vi "align.vi"(7 "I2C Ref Out":T1, 8 "error in (no error)":errorcluster, 11 "Angle":ext) -> (0 "error out":errorcluster, 2 "curAngle":ext, 3 "I2C Ref Out out":T1)   [LabVIEW 2017]
uses:
  <vilib>/myRIO/Instrument Drivers/Onboard IO/I2C/typedefs/I2C Reference.ctl
  <vilib>/myRIO/Common/Instrument Driver Framework/Utilities/typedefs/myRIO Generic Hardware Reference.ctl
  <vilib>/myRIO/Common/Instrument Driver Framework/Utilities/typedefs/Hardware Version Enum.ctl
  <vilib>/myRIO/Common/Instrument Driver Framework/Utilities/typedefs/myRIO v1.0 Reference.ctl
  <vilib>/myRIO/Common/Instrument Driver Framework/Utilities/typedefs/Generic FPGA Reference.ctl
  <vilib>/myRIO/Common/Instrument Driver Framework/myRIO v1.0/I2C/typedefs/I2C Channels Enum.ctl
  <vilib>/myRIO/Instrument Drivers/Onboard IO/I2C/typedefs/I2C Configuration.ctl
  <vilib>/myRIO/Instrument Drivers/Onboard IO/I2C/typedefs/I2C Transfer Rate.ctl
  <vilib>/myRIO/Instrument Drivers/Onboard IO/PWM/typedefs/PWM Reference.ctl
  <vilib>/myRIO/Common/Instrument Driver Framework/myRIO v1.0/PWM/typedefs/PWM Channels Enum.ctl
  <vilib>/myRIO/Instrument Drivers/Onboard IO/PWM/typedefs/PWM Configuration.ctl
  <vilib>/userdefined/High Color/nirio_resource_hc.ctl
  <vilib>/myRIO/Instrument Drivers/Onboard IO/DIO/typedefs/DIO Reference.ctl
  <vilib>/myRIO/Common/Instrument Driver Framework/myRIO v1.0/DIO/typedefs/DIO Channels List.ctl
  <vilib>/myRIO/Common/Instrument Driver Framework/myRIO v1.0/DIO/typedefs/DIO Channels Enum.ctl
  <vilib>/myRIO/Common/Instrument Driver Framework/Utilities/vis/Is FPGA Ref Available.vi
  <vilib>/myRIO/Common/Instrument Driver Framework/myRIO v1.0/PWM/vis/myRIO v1.1 Open PWM.vi
  <vilib>/myRIO/Instrument Drivers/Onboard IO/PWM/vis/Set Duty Cycle and Frequency.vi
  <vilib>/myRIO/Common/Instrument Driver Framework/myRIO v1.0/DIO/vis/myRIO v1.1 Open DIO.vi
  <vilib>/myRIO/Instrument Drivers/Onboard IO/DIO/vis/Write.vi
  <vilib>/myRIO/Common/Instrument Driver Framework/Utilities/vis/Validate Channels.vi
  <vilib>/myRIO/Common/Instrument Driver Framework/myRIO v1.0/PWM/vis/myRIO v1.0 Reserve PWM.vi
  <vilib>/myRIO/Common/Instrument Driver Framework/myRIO v1.0/DIO/vis/myRIO v1.0 Reserve DIO.vi
  <vilib>/myRIO/Common/Instrument Driver Framework/myRIO v1.0/PWM/vis/myRIO v1.0 Build MUX Configuration PWM.vi
  <vilib>/myRIO/Common/Instrument Driver Framework/myRIO v1.0/Resource Manager/vis/myRIO v1.0 Reserve Channel List.vi
  <vilib>/myRIO/Common/Instrument Driver Framework/myRIO v1.0/DIO/vis/myRIO v1.0 Build MUX Configuration DIO.vi
  <vilib>/myRIO/Common/Instrument Driver Framework/myRIO v1.0/Resource Manager/vis/myRIO v1.0 Create Configuration List.vi
  <vilib>/myRIO/Common/Instrument Driver Framework/myRIO v1.0/Resource Manager/vis/myRIO v1.0 Reserve Channel.vi
  <vilib>/myRIO/Common/Instrument Driver Framework/myRIO v1.0/Resource Manager/vis/myRIO v1.0 Unreserve Channel.vi
  <vilib>/myRIO/Common/Instrument Driver Framework/myRIO v1.0/Resource Manager/vis/myRIO v1.0 Build Mutex Name.vi
  <vilib>/Utility/VariantDataType/GetNumericInfo.vi
  <vilib>/Utility/error.llb/Error Cluster From Error Code.vi
  <vilib>/myRIO/Common/Instrument Driver Framework/myRIO v1.0/myRIO v1.1 Open.vi
  <vilib>/myRIO/Common/Instrument Driver Framework/Utilities/vis/IO Manager.vi
  <vilib>/myRIO/Common/Instrument Driver Framework/Utilities/vis/Configuration Manager.vi
  <vilib>/myRIO/Common/Instrument Driver Framework/myRIO v1.0/Resource Manager/vis/myRIO v1.0 Configure IO.vi
  <vilib>/myRIO/Common/Instrument Driver Framework/myRIO v1.0/myRIO v1.0 Close.vi
  <vilib>/myRIO/Common/Instrument Driver Framework/myRIO v1.0/DIO/vis/myRIO v1.0 Write DIO.vi
  <vilib>/myRIO/Common/Instrument Driver Framework/myRIO v1.0/PWM/vis/myRIO v1.0 Write PWM.vi
  <vilib>/myRIO/Express VI/Onboard IO/DO/DO Express VI.xnode
  <vilib>/myRIO/Instrument Drivers/Onboard IO/DIO/vis/myRIO DIO Open.xnode
  <vilib>/myRIO/Express VI/Onboard IO/PWM/PWM Express VI.xnode
  <vilib>/myRIO/Instrument Drivers/Onboard IO/PWM/vis/myRIO PWM Open.xnode
  <vilib>/myRIO/Instrument Drivers/Onboard IO/DIO/DIO.lvlib
  <vilib>/myRIO/Instrument Drivers/Onboard IO/PWM/PWM.lvlib
  <vilib>/myRIO/Instrument Drivers/Onboard IO/I2C/I2C.lvlib
panel:
  in  "stop":bool
  out "Aligned":bool
  in  "choosed":bool
  out "coerced angle":ext
  in  "R_PWM":dbl=0.5
  in  "L_PWM":dbl=0.5
  in  "range":ext=5.0 format="%#_13g"
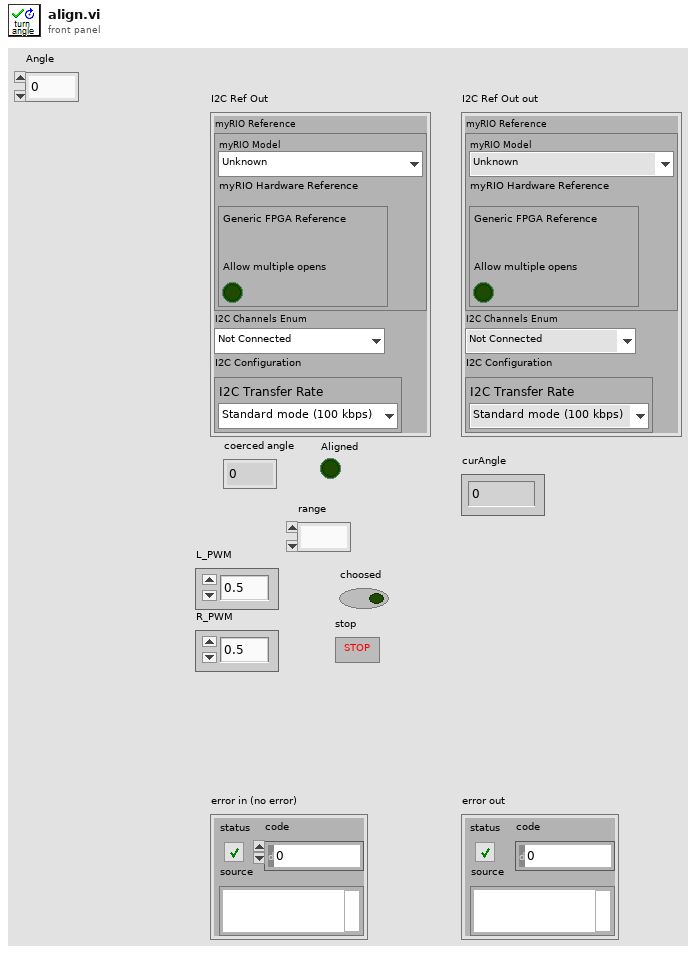
[diagram p1: front panel]
types:
  T1 = typedef "I2C.lvlib/I2C Reference.ctl" = cluster{"myRIO Reference":T2, "I2C Channels Enum":T6, "I2C Configuration":T7}
  T2 = typedef "myRIO Generic Hardware Reference.ctl" = cluster{"myRIO Model":T3, "myRIO Hardware Reference":T4}
  T3 = typedef "Hardware Version Enum.ctl" = enum16{"Unknown", "myRIO-1900", "myRIO-1950", "roboRIO", "NI ELVIS RIO CM"}
  T4 = typedef "myRIO v1.0 Reference.ctl" = cluster{"Generic FPGA Reference":T5, "Allow multiple opens":bool}
  T5 = typedef "Generic FPGA Reference.ctl" = refnum<k20>
  T6 = typedef "I2C Channels Enum.ctl" = enum16{"Not Connected", "A/I2C", "B/I2C", "I2C/I2C"}
  T7 = typedef "I2C.lvlib/I2C Configuration.ctl" = cluster{"I2C Transfer Rate":T8}
  T8 = typedef "I2C.lvlib/I2C Transfer Rate.ctl" = enum16{"Standard mode (100 kbps)", "Fast mode (400 kbps)"}
  T9 = typedef "DIO.lvlib/DIO Reference.ctl" = cluster{"myRIO Reference":T2, "DIO Channels List":T10}
  T10 = typedef "DIO Channels List.ctl" = T11[]
  T11 = typedef "DIO Channels Enum.ctl" = enum16{"Not Connected", "C/DIO0", "C/DIO1", "C/DIO2", "C/DIO3", "C/DIO4", "C/DIO5", "C/DIO6", "C/DIO7", "A/DIO0", "A/DIO1", "A/DIO2", "A/DIO3", "A/DIO4", "A/DIO5", "A/DIO6", "A/DIO7", "A/DIO8", "A/DIO9", "A/DIO10", "A/DIO11", "A/DIO12", "A/DIO13", "A/DIO14", "A/DIO15", "B/DIO0", "B/DIO1", "B/DIO2", "B/DIO3", "B/DIO4", "B/DIO5", "B/DIO6", "B/DIO7", "B/DIO8", "B/DIO9", "B/DIO10", "B/DIO11", "B/DIO12", "B/DIO13", "B/DIO14", "B/DIO15", "LED0", "LED1", "LED2", "LED3", "Button0", "DIO/DIO0", "DIO/DIO1", "DIO/DIO2", "DIO/DIO3", "DIO/DIO4", "DIO/DIO5", "DIO/DIO6", "DIO/DIO7", "DIO/DIO8", "DIO/DIO9", "SPI/CS0", "SPI/CS1", "SPI/CS2", "SPI/CS3", "LED RADIO (Green)", "LED RADIO (Red)", "LED COMM (Green)", "LED COMM (Red)", "LED MODE (Green)", "LED MODE (Red)"}
  T12 = typedef "nirio_resource_hc.ctl" = tag
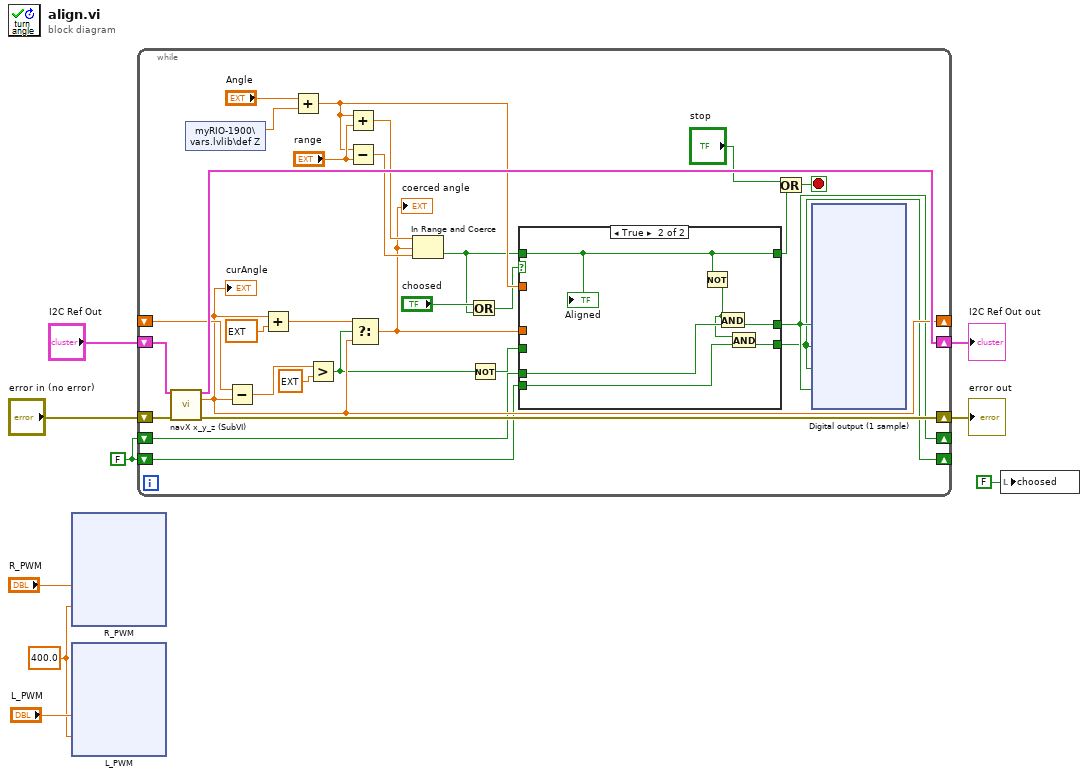
[diagram p0: block diagram]
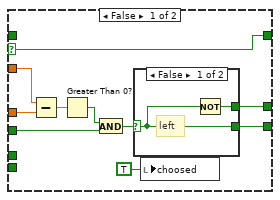
[diagram p2: hidden frame]
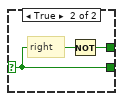
[diagram p3: hidden frame]
diagram:
  w2 = FALSE
  w3 = 400.0 ("Frequency [Hz]")
  n1 = xnode "R_PWM"("Duty Cycle"="R_PWM", "Frequency [Hz]"=w3) -> ()  [unwired: 1 in, 1 out]
  n2 = xnode "L_PWM"("Duty Cycle"="L_PWM", "Frequency [Hz]"=w3) -> ()  [unwired: 1 in, 1 out]
  n3 = while {
    shift-right: [w35] -> w6
    shift-left: "I2C Ref Out" -> [w38]
    shift-right: [w36] -> w7
    shift-left: "error in (no error)" -> [w37]
    shift-right: [w22] -> _
    shift-left: _ -> [w27]
    shift-right: [w15] -> _
    shift-left: w2 -> [w13]
    shift-right: [w14] -> _
    shift-left: w2 -> [w12]
    stop <- w11 stop-if-true
    n4 = call "navX x_y_z (SubVI).vi"("I2C Ref Out in"=w38, "error in (no error)"=w37) -> ("I2C Ref Out out"=w35:T1, "value Z"=w22:ext, "error out"=w36:errorcluster)  [unwired: 9 in, 2 out]
    "curAngle" <- w22
    n5 = shared-variable "myRIO-1900\\vars.lvlib\\def Z"() -> (w29:ext)  [unwired: 1 in, 1 out]
    n6 = Subtract(x=w27, y=w22) -> (x-y=w26:ext)
    n7 = Add(x=w22, y=ext 360.0) -> (x+y=w24:ext)
    n8 = Add(x="Angle", y=w29) -> (x+y=w30:ext)
    n9 = Greater?(x=w26, y=ext 20.0) -> (0:w20:bool)
    n10 = Add(x=w30, y="range") -> (x+y=w32:ext)
    n11 = Subtract(x=w30, y="range") -> (x-y=w33:ext)
    n12 = Select(t=w24, s=w20, f=w22) -> (s? t:f=w21:ext)
    "coerced angle" <- w21
    n13 = In Range and Coerce(upper limit=w32, x=w21, lower limit=w33) -> (In Range?=w16:bool)  [unwired: 1 out]
    n14 = Or(x="choosed", y=w16) -> (x .or. y?=w18:bool)
    n15 = Not(x=w20) -> (.not. x?=w19:bool)
    n16 = case shown="True" w18 {
      selector: w18 -> [w80 _]
      tunnel: [w84 w94] -> w15
      tunnel: [w83 w93] -> w14
      tunnel: w21 -> [w82 _]
      tunnel: w30 -> [w81 _]
      tunnel: [w80 w92] -> w28
      tunnel: w19 -> [w78 _]
      tunnel: w16 -> [_ w92]
      tunnel: w13 -> [_ w96]
      tunnel: w12 -> [_ w95]
      frame False {
        n17 = Subtract(x=w81, y=w82) -> (x-y=w85:ext)
        n18 = Greater Than 0?(x=w85) -> (x > 0?=w86:bool)
        n19 = And(x=w86, y=w78) -> (x .and. y?=w79:bool)
        n20 = case shown="False" w79 {
          selector: w79 -> [w88 w90]
          tunnel: [w87 w89] -> w84
          tunnel: [w88 w90] -> w83
          frame False {
            # "left"
            n21 = Not(x=w88) -> (.not. x?=w87:bool)
          }
          frame True {
            # "right"
            n22 = Not(x=w90) -> (.not. x?=w89:bool)
          }
        }
        n23 = local write "choosed"(TRUE ("choosed")) -> ()
      }
      frame True {
        n24 = Not(x=w92) -> (.not. x?=w91:bool)
        n25 = And(x=w91, y=w96) -> (x .and. y?=w94:bool)
        n26 = And(x=w91, y=w95) -> (x .and. y?=w93:bool)
        "Aligned" <- w92
      }
    }
    n27 = Or(x="stop", y=w28) -> (x .or. y?=w11:bool)
    n28 = xnode "Digital output (1 sample)"("Left+ (A/DIO5 (Pin 21))"=w15, "Right+ (A/DIO7 (Pin 25))"=w14, "Left- (A/DIO6 (Pin 23))"=w14, "Right- (A/DIO13 (Pin 26))"=w15) -> ()  [unwired: 1 in, 1 out]
  }
  "I2C Ref Out out" <- w6
  "error out" <- w7
  n29 = local write "choosed"(FALSE ("choosed")) -> ()
